vi "Logging.Start.vi"(8 "error in (no error)":errorcluster, 10 "NIVS.GatewayIPAddress":string, 11 "LogSpec":T1) -> (0 "error out":errorcluster, 2 "GUID":string, 3 "LogRef":T2)   [LabVIEW 2015, in "Single Station Execution.lvlib"]
uses:
  Single Station Execution.lvlib
  <vilib>/NI Veristand/Execution/DataLogging/IDataLogging Ref.ctl
  NationalInstruments.VeriStand.ClientAPI
  <vilib>/NI Veristand/Execution/DataLogging/DataLoggingSpecification Ref.ctl
  <vilib>/NI Veristand/Execution/DataLogging/NI_VS Data Logging API.lvlib
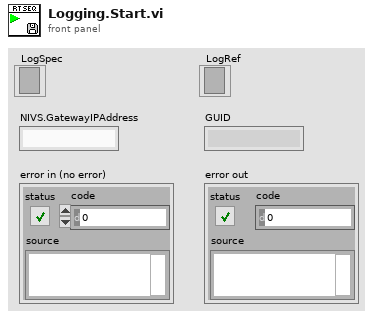
[diagram p1: front panel]
types:
  T1 = typedef "NI_VS Data Logging API.lvlib/DataLoggingSpecification Ref.ctl" = refnum<k24>
  T2 = typedef "NI_VS Data Logging API.lvlib/IDataLogging Ref.ctl" = refnum<k24>
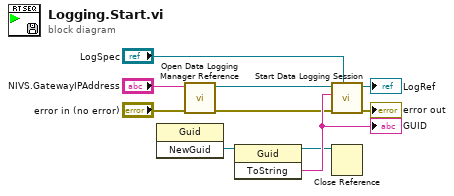
[diagram p0: block diagram]
diagram:
  n1 = invoke class="Guid" method="NewGuid"() -> ("NewGuid"=w8:refnum<k24>)  [unwired: 3 in, 2 out]
  n2 = call <vilib>:"Open Data Logging Manager Reference.vi"("error in (no error)"="error in (no error)", "Gateway IP Address (\"\": localhost)"="NIVS.GatewayIPAddress") -> ("error out"=w4:errorcluster, "Data Logging Manager Ref out"=w5:T2)  [unwired: 8 in]
  n3 = invoke class="Guid" method="ToString"(reference=w8) -> (reference out=w9:refnum<k24>, "ToString"=w10:string)  [unwired: 2 in, 1 out]
  "GUID" <- w10
  n4 = call <vilib>:"Start Data Logging Session.vi"("Data Logging Specification Ref in"="LogSpec", "error in (no error)"=w4, "Session Name in"=w10, "Data Logging Manager Ref in"=w5) -> ("error out"=→"error out":errorcluster, "Data Logging Manager Ref out"=→"LogRef":T2)  [unwired: 5 in, 1 out]
  n5 = Close Reference(reference=w9) -> ()  [unwired: 1 in, 1 out]
